vi "DrawSpotMap.vi"(3 "Draw Mode":u16(ring) items=["Frame", "Paint", "Invert Frame", "Invert Paint"], 4 "error in (no error)":errorcluster, 5 "radius":i32, 6 "Coefficients (2D)":sgl[][](array[numeric]) format="%.2f", 7 "Image Dst":T1) -> (0 "error out":errorcluster, 1 "Spot Map":T1)   [LabVIEW 2009]
uses:
  <vilib>/vision/Image Controls.llb/IMAQ Image.ctl
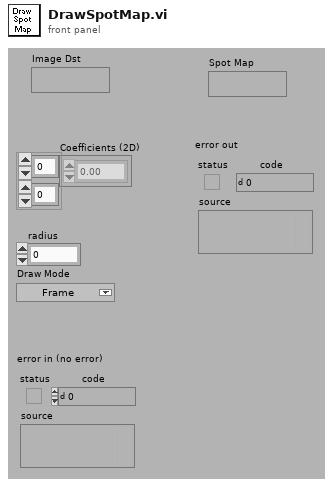
[diagram p1: front panel]
types:
  T1 = typedef "IMAQ Image.ctl" = refnum<image>
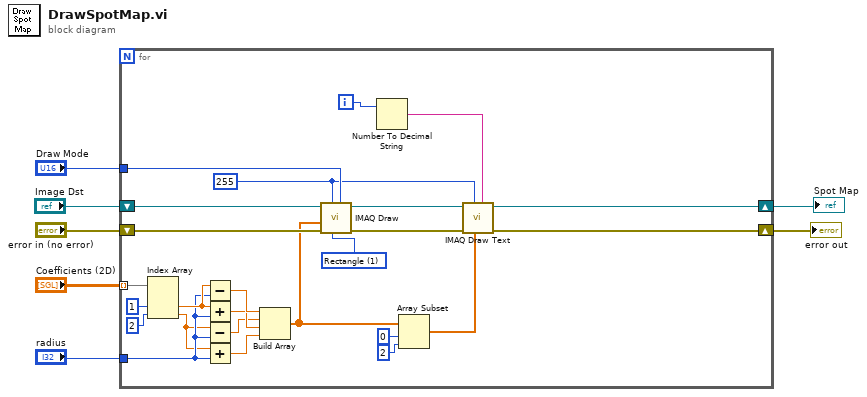
[diagram p0: block diagram]
diagram:
  n1 = for {
    tunnel: "Coefficients (2D)" -> [w32] mode=indexing
    shift-right: [w16] -> w5
    shift-left: "Image Dst" -> [w29]
    tunnel: "radius" -> [w25]
    tunnel: "Draw Mode" -> [w20]
    shift-right: [w8] -> w3
    shift-left: "error in (no error)" -> [w19]
    i -> [w13]
    w15 = 255
    w21 = u16 1 items=["Line", "Rectangle", "Oval"] ("Shape to draw")
    n2 = Index Array(array=w32, index #2=1 ("index"), index #3=2 ("index")) -> (element #2=w27:sgl, element #3=w24:sgl)  [unwired: 1 in, 1 out]
    n3 = Subtract(x=w27, y=w25) -> (x-y=w28:sgl)
    n4 = Add(x=w27, y=w25) -> (x+y=w26:sgl)
    n5 = Subtract(x=w24, y=w25) -> (x-y=w23:sgl)
    n6 = Add(x=w24, y=w25) -> (x+y=w22:sgl)
    n7 = Build Array(w28, w23, w26, w22) -> (w12:sgl[])
    n8 = call "IMAQ Draw"("Draw Mode"=w20, "Shape to draw"=w21, "Pixel Color"=w15, "error in (no error)"=w19, "Coordinates"=w12, "Image Src"=w29) -> ("error out"=w17:errorcluster, "Image Dst Out"=w18:T1)  [unwired: 4 in]
    n9 = Number To Decimal String(number=w13) -> (decimal integer string=w14:string)  [unwired: 1 in]
    n10 = Array Subset(array=w12, index=0, length=2) -> (w11:sgl[])
    n11 = call "IMAQ Draw Text"("String"=w14, "Insertion Point"=w11, "Color"=w15, "error in (no error)"=w17, "Image Src"=w18) -> ("error out"=w8:errorcluster, "Image Dst Out"=w16:T1)  [unwired: 3 in, 2 out]
  }
  "Spot Map" <- w5
  "error out" <- w3
